vi "QueueToCommand.vi"(3 "timeout":i32=1000, 4 "Stop Btn Pressed?":bool, 5 "ROS":T1={"topic port"=1236, "Node"="/labview", "topic"="/robot/head/command_head_nod", "type"="std_msgs/Bool", "node port"=7000, "error "={"status"=FALSE, "code"=0, "source"=""}, "Direction"=enum."Publisher", "APIs"=[], "Update (ms)"=1, "write queue"=1}) -> (0 "data":string, 1 "Queue log":string, 2 "Command":string)   [LabVIEW 2010]
uses:
  SubVIs/_ROSDirection.ctl
  SubVIs/_ROSControl.ctl
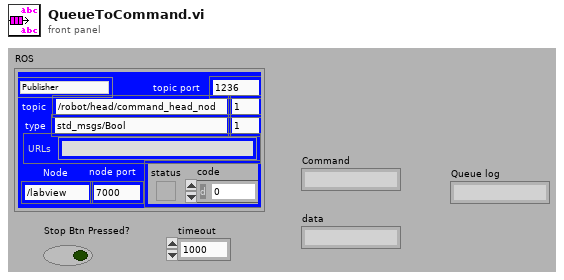
[diagram p1: front panel]
types:
  T1 = typedef "_ROSControl.ctl" = cluster{"topic port":u16, "Node":string, "topic":string, "type":string, "node port":u32, "error ":errorcluster, "Direction":T2, "APIs":string[], "Update (ms)":u16, "write queue":u16}
  T2 = typedef "_ROSDirection.ctl" = enum16{"Node", "Publisher", "Subscriber", "Service Client"}
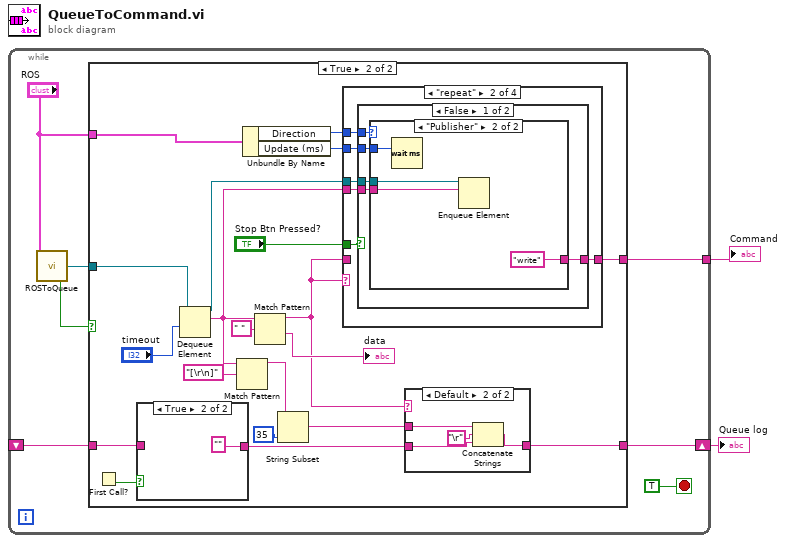
[diagram p0: block diagram]
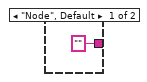
[diagram p4: hidden frame]
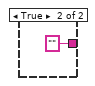
[diagram p5: hidden frame]
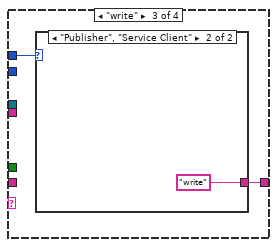
[diagram p6: hidden frame]
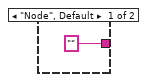
[diagram p7: hidden frame]
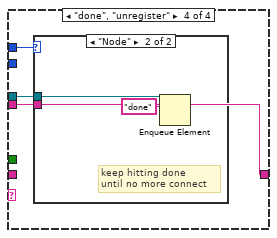
[diagram p8: hidden frame]
diagram:
  n1 = while {
    shift-right: [w9] -> w2
    shift-left: _ -> [w8]
    tunnel: [w4] -> w1
    stop <- TRUE stop-if-true
    n2 = call "ROSToQueue.vi"("ROS"="ROS") -> ("Available?"=w3:bool, "queue"=w6:refnum<queue>)  [unwired: 3 in]
    n3 = case shown="True" w3 {
      tunnel: [w10 w27] -> w9
      tunnel: w8 -> [w10 w25]
      tunnel: w6 -> [_ w19]
      tunnel: "ROS" -> [_ w18]
      tunnel: [_ w16] -> w4
      frame False {
      }
      frame True {
        n4 = First Call?() -> (First Call?: T/F=w28:bool)
        n5 = case shown="True" w28 {
          tunnel: [w63 "" ("regular expression")] -> w26
          tunnel: w25 -> [w63 _]
          frame False {
          }
          frame True {
          }
        }
        n6 = Dequeue Element(queue=w19, timeout in ms (-1)="timeout") -> (queue out=w20:refnum<queue>, element=w14:string)  [unwired: 1 in, 2 out]
        n7 = Match Pattern(string=w14, regular expression="[\r\n]") -> (before substring=w13:string)  [unwired: 1 in, 3 out]
        n8 = Unbundle By Name(w18) -> ("Direction"=w17:T2, "Update (ms)"=w11:u16)
        n9 = Match Pattern(string=w14, regular expression=" ") -> (before substring=w21:string, after substring=→"data":string)  [unwired: 1 in, 2 out]
        n10 = String Subset(string=w13, length (rest)=35 ("length (rest)")) -> (substring=w23:string)  [unwired: 1 in]
        n11 = case shown="\"repeat\"" w21 {
          tunnel: [w31 w35 w50 w53] -> w16
          tunnel: w21 -> [w31 _ _ _]
          tunnel: w20 -> [_ w37 _ w54]
          tunnel: w14 -> [_ w36 _ w53]
          tunnel: w17 -> [_ w34 w49 w55]
          tunnel: "Stop Btn Pressed?" -> [_ w33 _ _]
          tunnel: w11 -> [_ w32 _ _]
          frame Default {
          }
          frame "repeat" {
            n12 = case shown="False" w33 {
              tunnel: w37 -> [w42 _]
              tunnel: w36 -> [w41 _]
              tunnel: [w40 ""] -> w35
              tunnel: w34 -> [w39 _]
              tunnel: w32 -> [w38 _]
              frame False {
                n13 = case shown="\"Publisher\"" w39 {
                  tunnel: w42 -> [_ w47]
                  tunnel: w41 -> [_ w45]
                  tunnel: ["" "write"] -> w40
                  tunnel: w38 -> [_ w44]
                  frame "Node", Default {
                  }
                  frame "Publisher" {
                    n14 = Wait (ms)(milliseconds to wait=w44) -> ()  [unwired: 1 out]
                    n15 = Enqueue Element(queue=w47, element=w45) -> ()  [unwired: 2 in, 3 out]
                  }
                }
              }
              frame True {
              }
            }
          }
          frame "write" {
            n16 = case shown="\"Publisher\", \"Service Client\"" w49 {
              tunnel: ["" "write"] -> w50
              frame "Node", Default {
              }
              frame "Publisher", "Service Client" {
              }
            }
          }
          frame "done", "unregister" {
            n17 = case shown="\"Node\"" w55 {
              tunnel: w54 -> [_ w57]
              tunnel: w53 -> [_ _]
              frame Default {
              }
              frame "Node" {
                # "keep hitting done\nuntil no more connect"
                n18 = Enqueue Element(queue=w57, element="done") -> ()  [unwired: 2 in, 3 out]
              }
            }
          }
        }
        n19 = case shown="Default" w21 {
          tunnel: w26 -> [w58 w60]
          tunnel: [w58 w61] -> w27
          tunnel: w23 -> [_ w59]
          frame "" {
          }
          frame Default {
            n20 = Concatenate Strings(w59, "\r", w60) -> (w61:string)
          }
        }
      }
    }
  }
  "Queue log" <- w2
  "Command" <- w1
